vi "deg2rad (SubVI).vi"(1 "Angle [deg]":dbl) -> (0 "Angle[rad]":dbl)   [LabVIEW 2014]
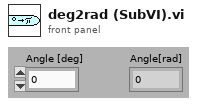
[diagram p1: front panel]
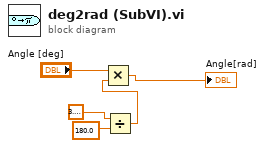
[diagram p0: block diagram]
diagram:
  n1 = Divide(x=3.141592653589793, y=180.0) -> (x/y=w2:dbl)
  n2 = Multiply(x="Angle [deg]", y=w2) -> (x*y=→"Angle[rad]":dbl)
